vi "Exercise2.5-DSB_RTL-SDR_RX-OK3.vi"() -> ()   [LabVIEW 2013]
uses:
  <vilib>/sound2/lvsound2.llb/Sound Data Format.ctl
  <vilib>/Analysis/2dsp.llb/Rational Resample (single channel, DBL).vi
  <vilib>/sound2/lvsound2.llb/Sound Output Write (DBL Single).vi
  rtlsdr/rtlsdr.lvlib
  <vilib>/Analysis/NI_AALPro.lvlib
panel:
  in  "Device index":u32
  out "Samples Acquired":u32
  out "# elements in queue":i32
  out "DevRefnum":u64
  out "Spectrum (FFT)":waveform(dbl)(graph)
  out "XY Graph":cdb[](graph)
  out "error out":errorcluster
  in  "sound format":T1={"sample rate (S/s)"=44100.0, "number of channels"=1, "bits per sample"=16}
  in  "stop":bool
  in  "Center frequency":u32=104300000
  in  "IQ rate":u32=286650
  out "error out":errorcluster
  # "DSB Receiver"
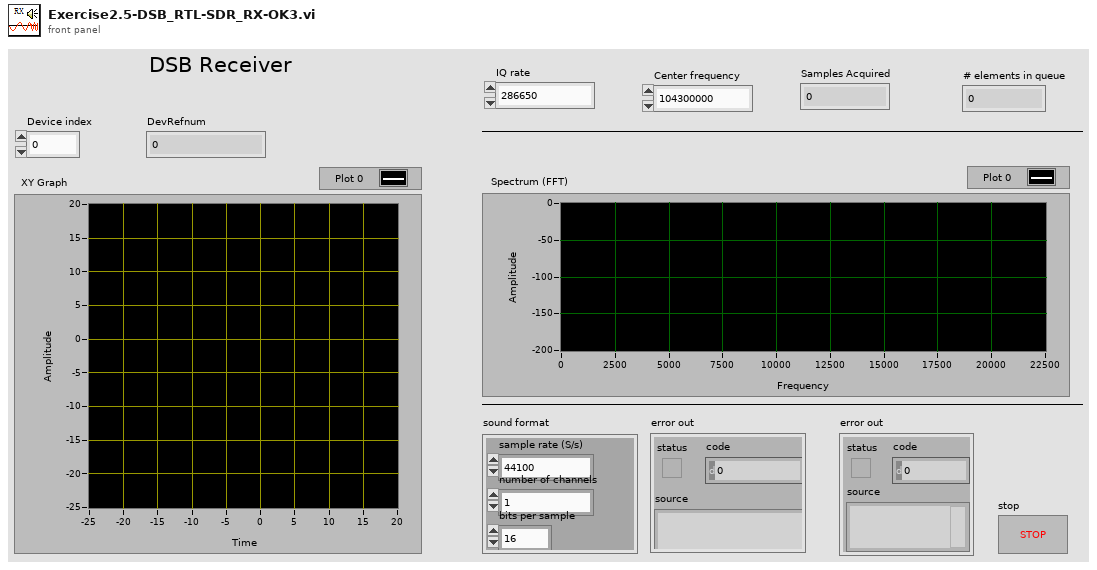
[diagram p1: front panel]
types:
  T1 = typedef "Sound Data Format.ctl" = cluster{"sample rate (S/s)":dbl, "number of channels":i32, "bits per sample":i32}
  T2 = typedef "Sound Output Task ID.ctl" = u32
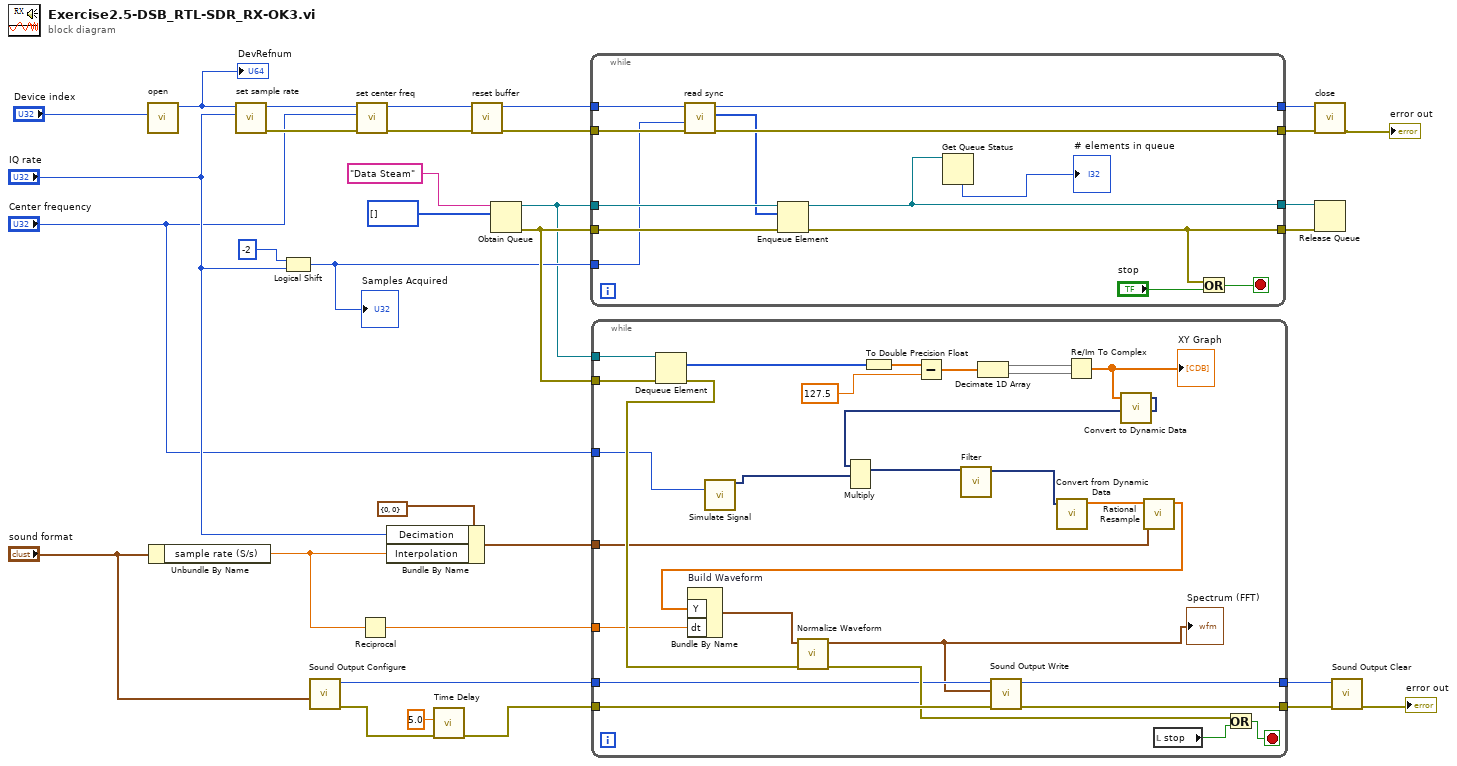
[diagram p0: block diagram]
diagram:
  n1 = call "open.vi"("index"="Device index") -> ("DevRefnum"=w26:u64)  [unwired: 9 in, 1 out]
  "DevRefnum" <- w26
  n2 = Unbundle By Name("sound format") -> ("sample rate (S/s)"=w2:dbl)
  n3 = call "set sample rate.vi"("rate"="IQ rate", "DevRefnum"=w26) -> ("error out"=w28:errorcluster, "DevRefnum"=w30:u64)  [unwired: 7 in, 1 out]
  n4 = Logical Shift(y=i16 -2, x="IQ rate") -> (x << y=w4:u32)
  "Samples Acquired" <- w4
  n5 = call <vilib>:"Sound Output Configure.vi"("sound format"="sound format") -> ("error out"=w9:errorcluster, "task ID"=w19:T2)  [unwired: 9 in]
  n6 = call "set center freq.vi"("error in (no error)"=w28, "freq"="Center frequency", "DevRefnum"=w30) -> ("error out"=w27:errorcluster, "DevRefnum"=w29:u64)  [unwired: 6 in, 1 out]
  n7 = Reciprocal(x=w2) -> (1/x=w12:dbl)
  n8 = Bundle By Name(cluster=cluster{"Interpolation":i32, "Decimation":i32} {"Interpolation"=0, "Decimation"=0}, "Decimation"="IQ rate", "Interpolation"=w2) -> (w11:cluster{"Interpolation":i32, "Decimation":i32})
  n9 = call "Time Delay"("error in (no error)"=w9, "Delay Time (s)"=5.0) -> ("error out"=w10:errorcluster)  [unwired: 9 in]
  n10 = call "reset buffer.vi"("error in (no error)"=w27, "DevRefnum"=w29) -> ("error out"=w24:errorcluster, "DevRefnum"=w25:u64)  [unwired: 8 in]
  n11 = Obtain Queue(name (unnamed)="Data Steam", element data type=u8[] [] ("buf 2")) -> (queue out=w3:refnum<queue>, error out=w5:errorcluster)  [unwired: 3 in, 1 out]
  n12 = while {
    tunnel: [w44] -> w22
    tunnel: w25 -> [w46]
    tunnel: w24 -> [w45]
    tunnel: [w43] -> w21
    tunnel: w4 -> [w34]
    tunnel: w3 -> [w41]
    tunnel: [w40] -> w15
    tunnel: w5 -> [w39]
    tunnel: [w37] -> w14
    stop <- w35 stop-if-true
    n13 = call "read sync.vi"("error in (no error)"=w45, "len"=w34, "DevRefnum"=w46) -> ("error out"=w43:errorcluster, "buf 2"=w38:u8[], "DevRefnum"=w44:u64)  [unwired: 6 in]
    n14 = Enqueue Element(queue=w41, element=w38, error in (no error)=w39) -> (queue out=w40:refnum<queue>, error out=w37:errorcluster)  [unwired: 1 in, 1 out]
    n15 = Get Queue Status(queue=w40) -> (# elements in queue=→"# elements in queue":i32)  [unwired: 2 in, 7 out]
    n16 = Or(x=w37, y="stop") -> (x .or. y?=w35:bool)
  }
  n17 = while {
    tunnel: w19 -> [w58]
    tunnel: [w68] -> w18
    tunnel: [w67] -> w17
    tunnel: w10 -> [w69]
    tunnel: w3 -> [w66]
    tunnel: w12 -> [w51]
    tunnel: w11 -> [w59]
    tunnel: w5 -> [w64]
    tunnel: "Center frequency" -> [w56]
    stop <- w60 stop-if-true
    n18 = Dequeue Element(queue=w66, error in (no error)=w64) -> (element=w65:u8[], error out=w63:errorcluster)  [unwired: 1 in, 2 out]
    n19 = call "Simulate Signal"("Frequency"=w56) -> ("Sine"=w53:dynamicdata)  [unwired: 13 in, 1 out]
    n20 = To Double Precision Float(number=w65) -> (double precision float=w74:dbl[])
    n21 = Subtract(x=w74, y=127.5) -> (x-y=w72:dbl[])
    n22 = Decimate 1D Array "Decimate 1D Array"(w72) -> (w70:dbl[], w71:dbl[])
    n23 = Re/Im To Complex(1:w71, 2:w70) -> (0:w55:cdb[])
    "XY Graph" <- w55
    n24 = call "Convert to Dynamic Data"("Array"=w55) -> ("Dynamic Data Type"=w54:dynamicdata)  [unwired: 3 in]
    n25 = Multiply(1:w53, 2:w54) -> (0:w52:dynamicdata)  [unwired: 1 in, 1 out]
    n26 = call "Filter"("Signal"=w52) -> ("Filtered Signal"=w48:dynamicdata)  [unwired: 9 in, 1 out]
    n27 = call "Convert from Dynamic Data"("Dynamic Data Type"=w48) -> ("Array"=w49:dbl[])  [unwired: 3 in]
    n28 = call-poly <vilib>:"Rational Resample.vi"("resample factor"=w59, "X"=w49) -> ("Y"=w47:dbl[])  [unwired: 7 in, 2 out]
    n29 = Bundle By Name "Build Waveform"("Y"=w47, "dt"=w51) -> (w50:waveform(dbl))  [unwired: 1 in]
    n30 = call <vilib>:"Normalize Waveform.vi"("error in (no error)"=w63, "waveform in"=w50) -> ("error out"=w62:errorcluster, "normalized waveform"=w57:waveform(dbl))  [unwired: 6 in, 2 out]
    "Spectrum (FFT)" <- w57
    n31 = call-poly <vilib>:"Sound Output Write.vi"("error in (no error)"=w69, "data"=w57, "task ID"=w58) -> ("error out"=w67:errorcluster, "task ID out"=w68:T2)  [unwired: 7 in]
    n32 = local read "stop"() -> (w61:bool)
    n33 = Or(x=w62, y=w61) -> (x .or. y?=w60:bool)
  }
  n34 = call "close.vi"("error in (no error)"=w21, "DevRefnum"=w22) -> ("error out"=→"error out":errorcluster)  [unwired: 8 in, 1 out]
  n35 = Release Queue(queue=w15, error in (no error)=w14) -> ()  [unwired: 1 in, 3 out]
  n36 = call <vilib>:"Sound Output Clear.vi"("error in (no error)"=w17, "task ID"=w18) -> ("error out"=→"error out":errorcluster)  [unwired: 9 in]
